vi "Broadcast Origin.vi"(8 "error in (no error)":errorcluster, 11 "Map Model in":refnum<class "Map Model.lvclass">) -> (0 "error out":errorcluster, 3 "Map Model out":refnum<class "Map Model.lvclass">)   [LabVIEW 2020, in "Map Model.lvlib" / "Map Model.lvclass"]
uses:
  Map Model.lvclass
  Yaml Model/Yaml Model Messages/Abstract Origin Msg/Abstract Origin Msg.lvclass
  C:/Program Files/National Instruments/LabVIEW 2020/vi.lib/ActorFrameworkObserver/Data Message/Data Message.lvclass
  Map Model.lvclass/Map Model.ctl
  <vilib>/ActorFrameworkObserver/Actor Register/Actor Register.lvclass
panel:
  # "NOTICE -- YOU MUST LEAVE THIS NOTICE IN PLACE.\n\nCopyright (c) 2017, LIANG LIU Shawn.Liu.cn@gmail.com\nAll rights reserved.\n\nRedistribution and use in source and binary forms, with or without modification, are permitted provided that the following conditions are met:\n-Redistributions of source code must retain the above copyright notice, this list of conditions and the following disclaimer.\n-Redistributions in binary form must reproduce the above copyright notice, this list of conditions and the following disclaimer in the documentation and/or other materials provided with the distribution.\n-Neither the name of the eLp nor the names of its contributors may be used to endorse or promote products derived from this software without specific prior written permission.\n\nTHIS SOFTWARE IS PROVIDED BY THE COPYRIGHT HOLDERS AND CONTRIBUTORS \"AS IS\" AND ANY EXPRESS OR IMPLIED WARRANTIES, INCLUDING, BUT NOT LIMITED TO, THE IMPLIED WARRANTIES OF MERCHANTABILITY AND FITNESS FOR A PARTICULAR PURPOSE ARE DISCLAIMED. IN NO EVENT SHALL THE COPYRIGHT HOLDER OR CONTRIBUTORS BE LIABLE FOR ANY DIRECT, INDIRECT, INCIDENTAL, SPECIAL, EXEMPLARY, OR CONSEQUENTIAL DAMAGES (INCLUDING, BUT NOT LIMITED TO, PROCUREMENT OF SUBSTITUTE GOODS OR SERVICES; LOSS OF USE, DATA, OR PROFITS; OR BUSINESS INTERRUPTION) HOWEVER CAUSED AND ON ANY THEORY OF LIABILITY, WHETHER IN CONTRACT, STRICT LIABILITY, OR TORT (INCLUDING NEGLIGENCE OR OTHERWISE) ARISING IN ANY WAY OUT OF THE USE OF THIS SOFTWARE, EVEN IF ADVISED OF THE POSSIBILITY OF SUCH DAMAGE."
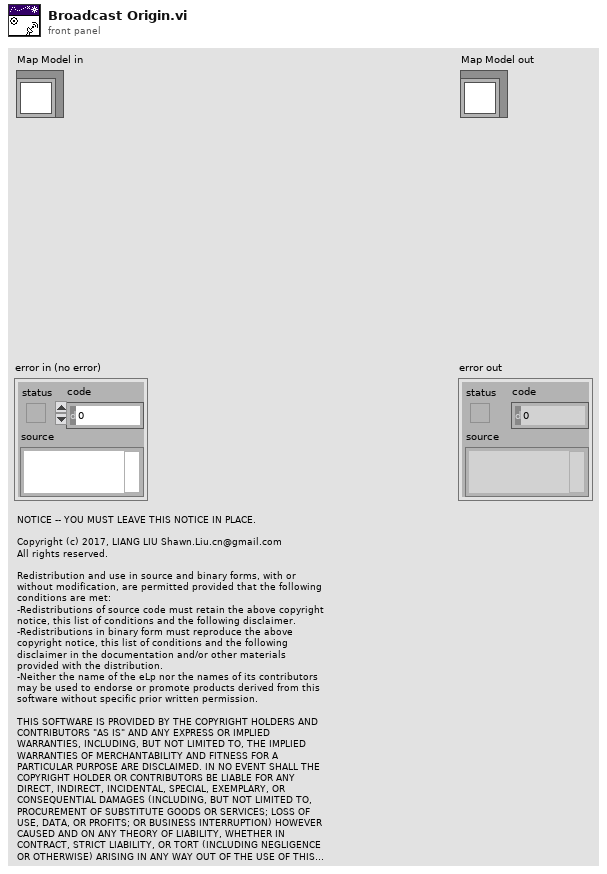
[diagram p1: front panel]
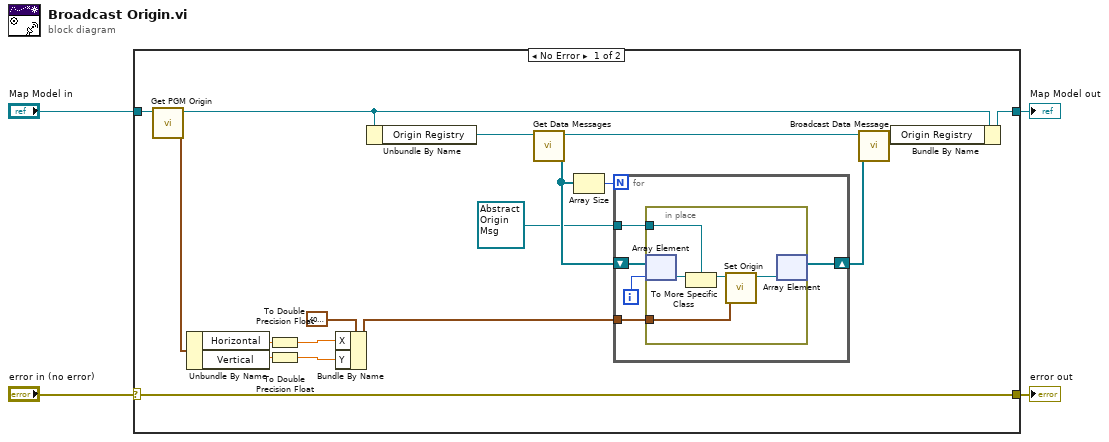
[diagram p0: block diagram]
diagram:
  n1 = case "Error Case" shown="No Error" "error in (no error)" {
    selector: "error in (no error)" -> [w14 w34]
    tunnel: "Map Model in" -> [w22 w33]
    tunnel: [w5 w33] -> w3
    tunnel: [w14 w34] -> w2
    frame No Error {
      n2 = call "Get PGM Origin.vi"("Map Model in"=w22) -> ("PGM Origin"=w10:cluster{"Horizontal":dbl, "Vertical":dbl}, "Map Model out"=w13:refnum<class "Map Model.lvclass">)  [unwired: 9 in]
      n3 = Unbundle By Name(w10) -> ("Horizontal"=w9:dbl, "Vertical"=w8:dbl)
      n4 = To Double Precision Float(number=w9) -> (double precision float=w7:dbl)
      n5 = To Double Precision Float(number=w8) -> (double precision float=w6:dbl)
      n6 = Bundle By Name(cluster=cluster{"X":dbl, "Y":dbl, "R":dbl} {"X"=0.0, "Y"=0.0, "R"=0.0} ("Origin"), "X"=w7, "Y"=w6) -> (w12:cluster{"X":dbl, "Y":dbl, "R":dbl})
      n7 = Unbundle By Name(w13) -> ("Origin Registry"=w21:refnum<class "Actor Register.lvclass">)
      n8 = call-dynamic "Get Data Messages.vi"("Actor Register in"=w21) -> ("Data Messages"=w18:refnum<class "Data Message.lvclass">[], "Actor Register out"=w20:refnum<class "Actor Register.lvclass">)  [unwired: 9 in]
      n9 = Array Size(array=w18) -> (size(s)=w16:i32)
      n10 = for {
        N: w16 -> [_]
        shift-right: [w25] -> w15
        shift-left: w18 -> [w27]
        tunnel: refnum<class "Abstract Origin Msg.lvclass"> refnum ("Yaml Model.lvlib:Abstract Origin Msg.lvclass") -> [w26]
        tunnel: w12 -> [w23]
        i -> [w24]
        n11 = in-place {
          in-place-border: w26 -> [w31]
          in-place-border: w23 -> [w28]
          n12 = in-place-array #1(w27, w24) -> (w32:refnum<class "Data Message.lvclass">)
          n13 = To More Specific Class(target class=w31, reference=w32) -> (specific class reference=w30:refnum<class "Abstract Origin Msg.lvclass">)  [unwired: 1 in, 1 out]
          n14 = call "Set Origin.vi"("Origin"=w28, "Abstract Origin Msg in"=w30) -> ("Abstract Origin Msg out"=w29:refnum<class "Abstract Origin Msg.lvclass">)  [unwired: 9 in]
          n15 = in-place-array #1(w29) -> (w25:refnum<class "Data Message.lvclass">[])  [unwired: 1 out]
        }
      }
      n16 = call <vilib>:"Broadcast Data Message.vi"("Data Messages"=w15, "Actor Register in"=w20) -> ("Actor Register out"=w19:refnum<class "Actor Register.lvclass">)  [unwired: 8 in, 1 out]
      n17 = Bundle By Name(cluster=w13, "Origin Registry"=w19) -> (w5:refnum<class "Map Model.lvclass">)
    }
    frame Error {
    }
  }
  "error out" <- w2
  "Map Model out" <- w3
